vi "rev_1D_tipconvolution.vi"() -> ()   [LabVIEW 2017]
panel:
  in  "stop":bool
  in  "angle":dbl=35.0 min=1.0 max=89.0 format="%.2f"
  in  "radius of curvature":dbl=50.0 min=1.0 max=1000.0 format="%.2f"
  in  "height":dbl=120.0 format="%.2f"
  in  "scanning speed":u32(slide)=66 scale=1.0..1000.0
  in  "slope":dbl=1.0 format="%.2f"
  out "Waveform Graph":dbl[][](graph)
  in  "width":dbl=140.0 format="%.2f"
  in  "period":dbl=310.0 format="%.2f"
  # "tipdefinition"
  # "sampleshape"
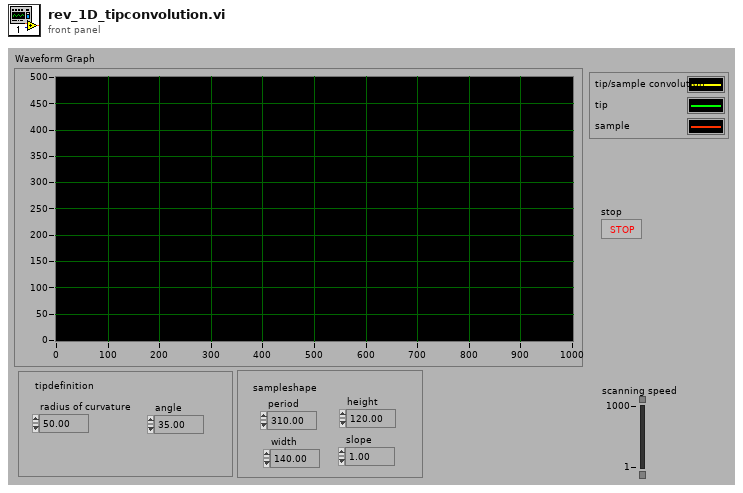
[diagram p1: front panel]
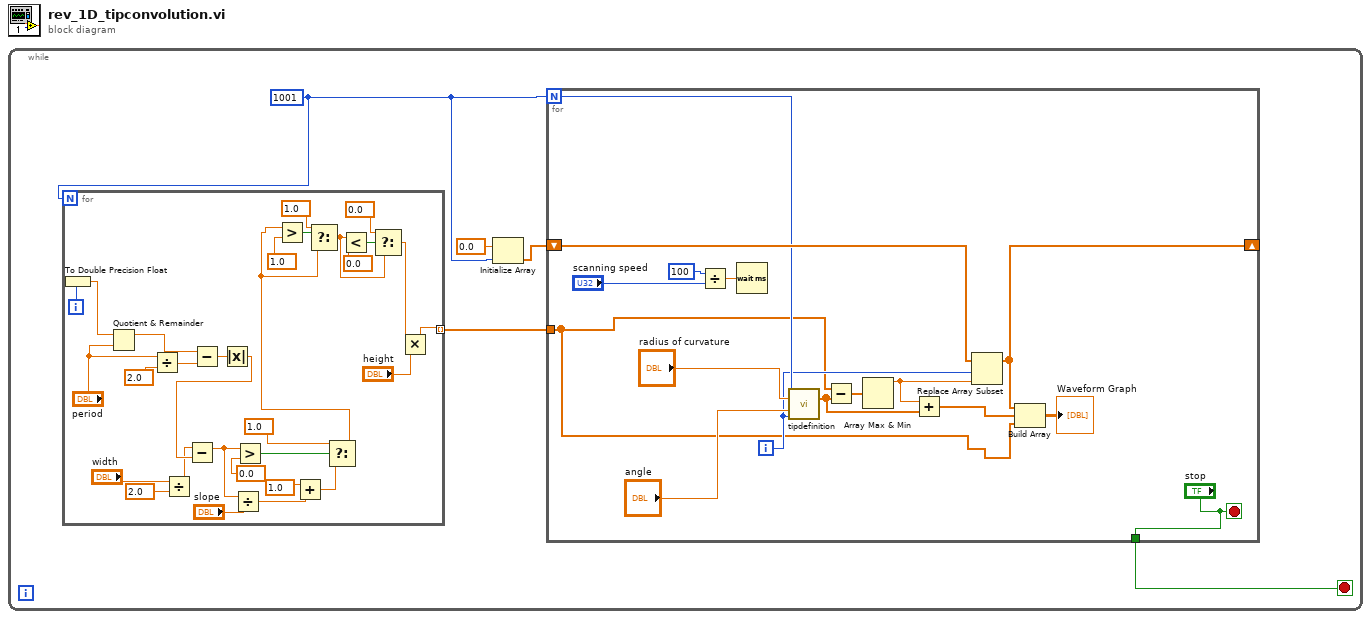
[diagram p0: block diagram]
diagram:
  n1 = while {
    stop <- w2 stop-if-true
    w1 = 1001
    n2 = for {
      N: w1 -> [_]
      tunnel: [w23] -> w5 mode=indexing
      i -> [w51]
      n3 = To Double Precision Float(number=w51) -> (double precision float=w22:dbl)
      n4 = Quotient & Remainder(x=w22, y="period") -> (x-y*floor(x/y)=w40:dbl)  [unwired: 1 out]
      n5 = Divide(x="period", y=2.0) -> (x/y=w39:dbl)
      n6 = Divide(x="width", y=2.0) -> (x/y=w35:dbl)
      n7 = Subtract(x=w40, y=w39) -> (x-y=w38:dbl)
      n8 = Absolute Value(x=w38) -> (abs(x)=w36:dbl)
      n9 = Subtract(x=w35, y=w36) -> (x-y=w29:dbl)
      n10 = Divide(x=w29, y="slope") -> (x/y=w28:dbl)
      n11 = Greater?(x=w29, y=0.0) -> (0:w33:bool)
      n12 = Add(x=1.0, y=w28) -> (x+y=w27:dbl)
      n13 = Select(t=1.0, s=w33, f=w27) -> (s? t:f=w26:dbl)
      n14 = Greater?(x=w26, y=1.0) -> (0:w46:bool)
      n15 = Select(t=1.0, s=w46, f=w26) -> (s? t:f=w41:dbl)
      n16 = Less?(x=w41, y=0.0) -> (x < y?=w43:bool)
      n17 = Select(t=0.0, s=w43, f=w41) -> (s? t:f=w24:dbl)
      n18 = Multiply(x=w24, y="height") -> (x*y=w23:dbl)
    }
    n19 = Initialize Array(0.0 ("Element Data"), w1) -> (w4:dbl[])
    n20 = for {
      N: w1 -> [w11]
      tunnel: w5 -> [w6]
      shift-right: [w20] -> _
      shift-left: w4 -> [w21]
      tunnel: ["stop"] -> w2
      i -> [w8]
      stop <- "stop" stop-if-true
      n21 = Divide(x=u32 100, y="scanning speed") -> (x/y=w18:dbl)
      n22 = Wait (ms)(milliseconds to wait=w18) -> ()  [unwired: 1 out]
      n23 = call "tipdefinition.vi"("#points"=w11, "radius of curvature"="radius of curvature", "tipangle"="angle", "offset"=w8) -> ("output"=w10:dbl[])  [unwired: 11 in]
      n24 = Subtract(x=w6, y=w10) -> (x-y=w9:dbl[])
      n25 = Array Max & Min(array=w9) -> (max value=w15:dbl)  [unwired: 3 out]
      n26 = Add(x=w15, y=w10) -> (x+y=w7:dbl[])
      n27 = Replace Array Subset(array=w21, new element=w15, index=w8) -> (w20:dbl[])
      n28 = Build Array(w20, w7, w6) -> (→"Waveform Graph":dbl[][])
    }
  }
